vi "Readout File Properties, Filtered.vi"(10 "Filter Type":T1=enum."Prealloc Clones", 11 "Selected Folder":path) -> (0 "error IO":errorcluster, 3 "Files":T2[](array[typedef]))   [LabVIEW 2022 SP3]
uses:
  TDs/FileProps.ctl
  TDs/PropToFilter.ctl
panel:
  out "VI: Num of Filtered":u16
  out "VI: Num of Files":u16
  out "VI: Current Idx":u16
  out "Num Of Folders":i32
  out "All Folders":path[](array[path])
  in  "Stop":bool
  out "Folder: Num of Files":i32
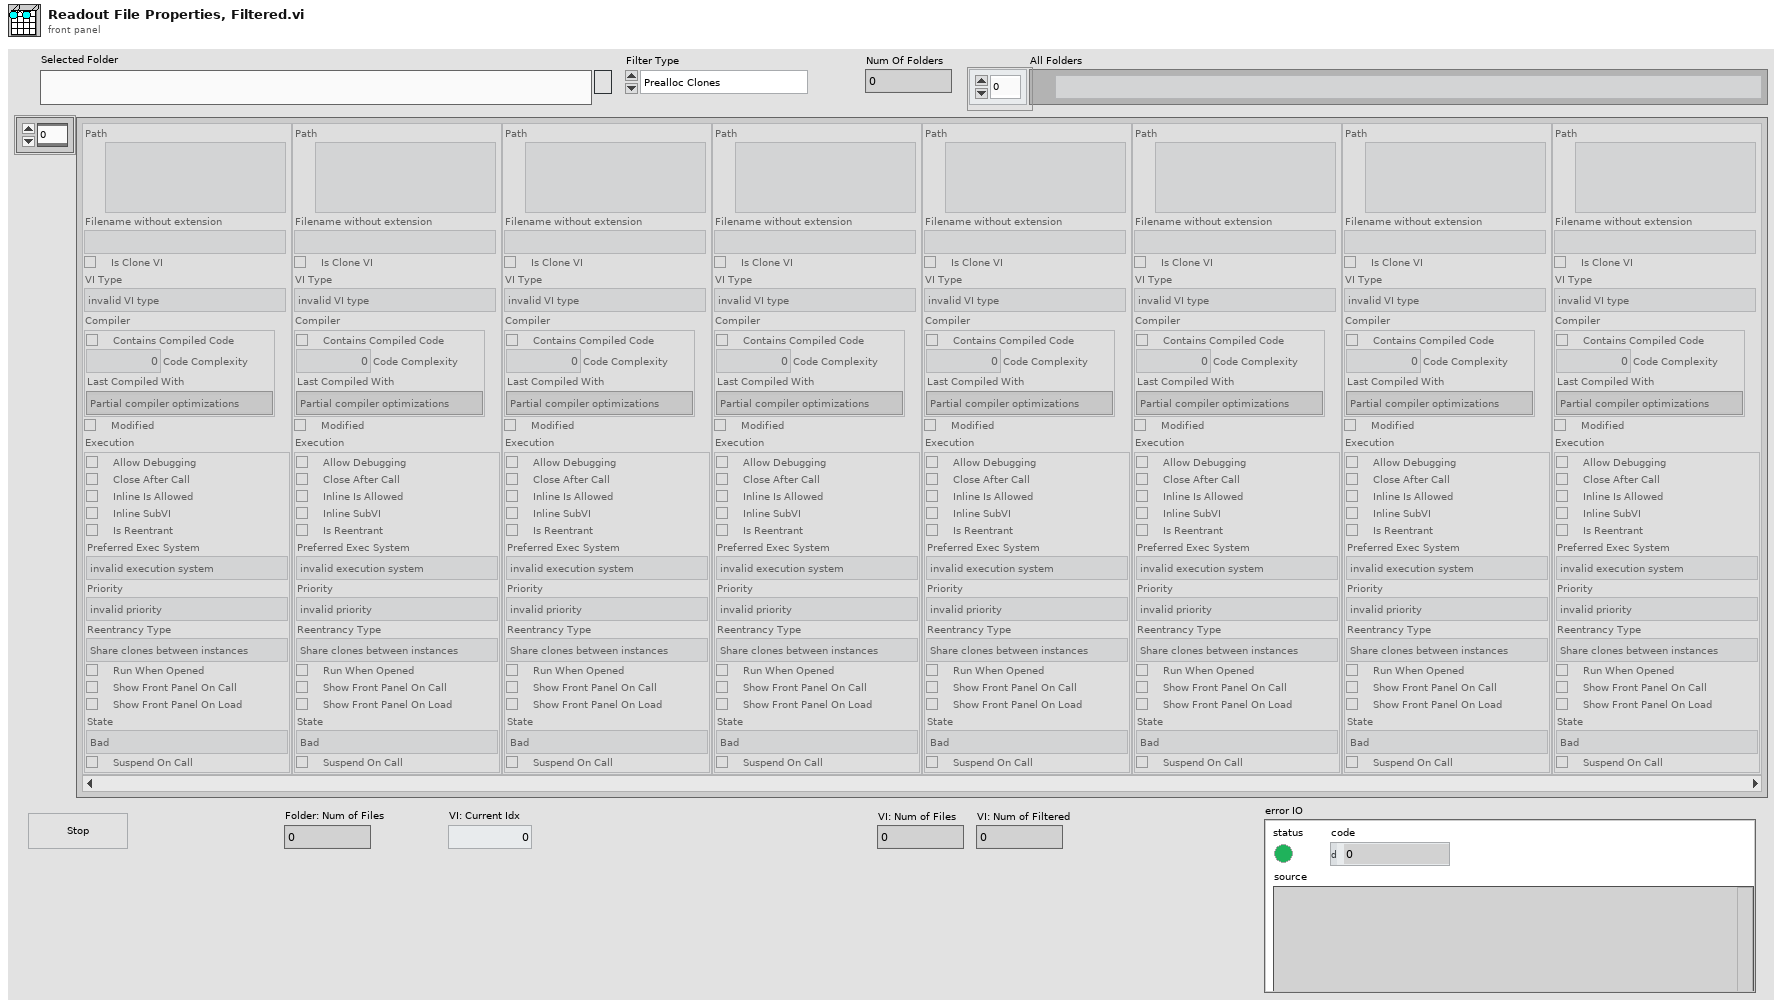
[diagram p1: front panel]
types:
  T1 = typedef "PropToFilter.ctl" = enum16{"None", "Prealloc Clones", "Separated Compiled Code", "Not Sep Compiled Code", "Modified"}
  T2 = typedef "FileProps.ctl" = cluster{"Path":path, "Filename without extension":string, "Is Clone VI":bool, "VI Type":enum32{"invalid VI type", "Standard VI", "Control VI", "Global VI", "Polymorphic VI", "Configuration VI", "SubSystem", "Facade VI", "Method VI", "Statechart Diagram VI"}, "Compiler":cluster{"Contains Compiled Code":bool, "Code Complexity":sgl, "Last Compiled With":enum16{"Partial compiler optimizations", "Full compiler optimizations"}}, "Modified":bool, "Execution":cluster{"Allow Debugging":bool, "Close After Call":bool, "Inline Is Allowed":bool, "Inline SubVI":bool, "Is Reentrant":bool, "Preferred Exec System":enum32{"invalid execution system", "user interface", "standard", "instrument i/o", "data acquisition", "other 1", "other 2", "same as caller"}, "Priority":enum32{"invalid priority", "background priority", "normal priority", "above normal priority", "high priority", "time critical priority", "subroutine"}, "Reentrancy Type":enum16{"Share clones between instances", "Preallocate clone for each instance"}, "Run When Opened":bool, "Show Front Panel On Call":bool, "Show Front Panel On Load":bool, "State":enum32{"Bad", "Idle", "Run top level", "Running"}, "Suspend On Call":bool}}
  T3 = enum16{"Share clones between instances", "Preallocate clone for each instance"}
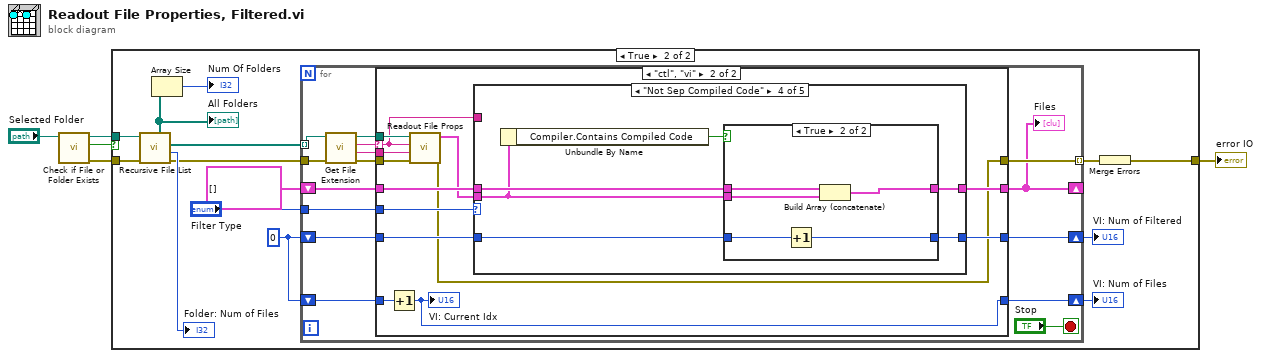
[diagram p0: block diagram]
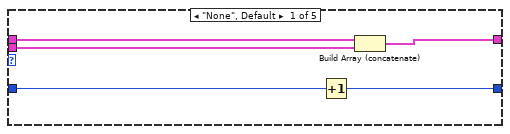
[diagram p4: hidden frame]
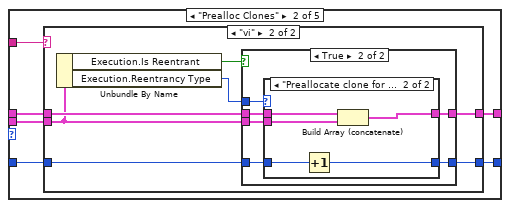
[diagram p5: hidden frame]
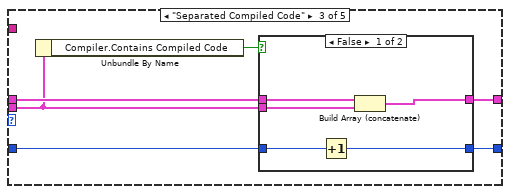
[diagram p9: hidden frame]
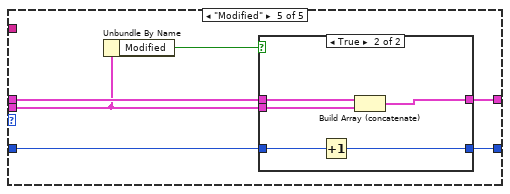
[diagram p12: hidden frame]
diagram:
  n1 = call <vilib>:"Check if File or Folder Exists.vi"("path"="Selected Folder") -> ("error out"=w2:errorcluster, "file or folder exists?"=w5:bool, "dup path"=w4:path)  [unwired: 8 in]
  n2 = case shown="True" w5 {
    tunnel: w4 -> [_ w19]
    tunnel: w2 -> [w6 w20]
    tunnel: [w6 w14] -> w1
    frame False {
    }
    frame True {
      w10 = u16 0 ("Current Idx")
      n3 = call <vilib>:"Recursive File List.vi"("error in (no error)"=w20, "Folder Path"=w19) -> ("error out"=w16:errorcluster, "Number of Files"=→"Folder: Num of Files":i32, "All Files in Dir"=w18:path[], "All Folders"=w13:path[])  [unwired: 5 in, 1 out]
      "All Folders" <- w13
      n4 = Array Size(array=w13) -> (size(s)=→"Num Of Folders":i32)
      n5 = for {
        tunnel: w18 -> [w34] mode=indexing
        tunnel: w16 -> [w33]
        tunnel: [w28] -> w15 mode=indexing
        shift-right: [w26] -> w9
        shift-left: w10 -> [w27]
        shift-right: [w24] -> _
        shift-left: T2[] [] -> [w25]
        shift-right: [w23] -> w8
        shift-left: w10 -> [w22]
        tunnel: "Filter Type" -> [w21]
        stop <- "Stop" stop-if-true
        n6 = call <vilib>:"Get File Extension.vi"("error in (no error)"=w33, "file"=w34) -> ("error out"=w32:errorcluster, "filename without extension"=w29:string, "lowercase file extension"=w30:string, "dup file"=w31:path)  [unwired: 5 in, 1 out]
        n7 = case shown="\"ctl\", \"vi\"" w30 {
          selector: w30 -> [_ w41]
          tunnel: w32 -> [w39 w45]
          tunnel: w31 -> [_ w44]
          tunnel: [w39 w43] -> w28
          tunnel: [w37 w50] -> w24
          tunnel: w29 -> [_ w40]
          tunnel: w27 -> [w38 w52]
          tunnel: [w38 w51] -> w26
          tunnel: w25 -> [w37 w49]
          tunnel: [w36 w48] -> w23
          tunnel: w22 -> [w36 w47]
          tunnel: w21 -> [_ w46]
          frame Default {
          }
          frame "ctl", "vi" {
            n8 = Increment(x=w52) -> (x+1=w51:u16)
            "VI: Current Idx" <- w51
            n9 = call "Readout File Props.vi"("error in (no error)"=w45, "filename without extension"=w40, "extension"=w41, "file path"=w44) -> ("error out"=w43:errorcluster, "Exec"=w42:T2)  [unwired: 6 in]
            n10 = case shown="\"Not Sep Compiled Code\"" w46 {
              tunnel: [w57 w63 w93 w106 w119] -> w50
              tunnel: w49 -> [w56 w62 w92 w105 w118]
              tunnel: [w55 w61 w91 w104 w117] -> w48
              tunnel: w47 -> [w54 w60 w90 w103 w116]
              tunnel: w42 -> [w53 w59 w89 w102 w115]
              tunnel: w41 -> [_ w58 _ _ _]
              frame "None", Default {
                n11 = Increment(x=w54) -> (x+1=w55:u16)
                n12 = Build Array (concatenate)(w56, w53) -> (w57:T2[])
              }
              frame "Prealloc Clones" {
                n13 = case shown="\"vi\"" w58 {
                  tunnel: [w65 w72] -> w63
                  tunnel: w62 -> [w65 w71]
                  tunnel: [w64 w69] -> w61
                  tunnel: w60 -> [w64 w68]
                  tunnel: w59 -> [_ w66]
                  frame Default {
                  }
                  frame "vi" {
                    n14 = Unbundle By Name(w66) -> ("Execution.Is Reentrant"=w67:bool, "Execution.Reentrancy Type"=w70:T3)
                    n15 = case shown="True" w67 {
                      tunnel: [w74 w80] -> w72
                      tunnel: w71 -> [w74 w79]
                      tunnel: w66 -> [_ w78]
                      tunnel: w70 -> [_ w77]
                      tunnel: [w73 w76] -> w69
                      tunnel: w68 -> [w73 w75]
                      frame False {
                      }
                      frame True {
                        n16 = case shown="\"Preallocate clone for each instance\"" w77 {
                          tunnel: [w82 w87] -> w80
                          tunnel: w79 -> [w82 w86]
                          tunnel: w78 -> [_ w85]
                          tunnel: [w81 w83] -> w76
                          tunnel: w75 -> [w81 w84]
                          frame "Share clones between instances", Default {
                          }
                          frame "Preallocate clone for each instance" {
                            n17 = Increment(x=w84) -> (x+1=w83:u16)
                            n18 = Build Array (concatenate)(w86, w85) -> (w87:T2[])
                          }
                        }
                      }
                    }
                  }
                }
              }
              frame "Separated Compiled Code" {
                n19 = Unbundle By Name(w89) -> ("Compiler.Contains Compiled Code"=w88:bool)
                n20 = case shown="False" w88 {
                  tunnel: [w98 w100] -> w93
                  tunnel: w92 -> [w97 w100]
                  tunnel: w89 -> [w96 _]
                  tunnel: [w95 w99] -> w91
                  tunnel: w90 -> [w94 w99]
                  frame False {
                    n21 = Increment(x=w94) -> (x+1=w95:u16)
                    n22 = Build Array (concatenate)(w97, w96) -> (w98:T2[])
                  }
                  frame True {
                  }
                }
              }
              frame "Not Sep Compiled Code" {
                n23 = Unbundle By Name(w102) -> ("Compiler.Contains Compiled Code"=w101:bool)
                n24 = case shown="True" w101 {
                  tunnel: [w108 w113] -> w106
                  tunnel: w105 -> [w108 w112]
                  tunnel: w102 -> [_ w111]
                  tunnel: [w107 w110] -> w104
                  tunnel: w103 -> [w107 w109]
                  frame False {
                  }
                  frame True {
                    n25 = Increment(x=w109) -> (x+1=w110:u16)
                    n26 = Build Array (concatenate)(w112, w111) -> (w113:T2[])
                  }
                }
              }
              frame "Modified" {
                n27 = Unbundle By Name(w115) -> ("Modified"=w114:bool)
                n28 = case shown="True" w114 {
                  tunnel: [w121 w126] -> w119
                  tunnel: w118 -> [w121 w125]
                  tunnel: w115 -> [_ w124]
                  tunnel: [w120 w123] -> w117
                  tunnel: w116 -> [w120 w122]
                  frame False {
                  }
                  frame True {
                    n29 = Increment(x=w122) -> (x+1=w123:u16)
                    n30 = Build Array (concatenate)(w125, w124) -> (w126:T2[])
                  }
                }
              }
            }
          }
        }
        "Files" <- w24
      }
      "VI: Num of Files" <- w9
      "VI: Num of Filtered" <- w8
      n31 = Merge Errors(w15) -> (w14:errorcluster)
    }
  }
  "error IO" <- w1
